vi "TIFFStream Write.vi"(7 "File data":T1, 8 "error in (no error)":errorcluster, 9 "Last image in file?":bool, 10 "Current and next IFD offset in":u32[](array[numeric]), 11 "Image data reference":refnum<data-value>) -> (0 "error out":errorcluster, 2 "Current and next IFD offset out":u32[](array[numeric]), 5 "File data out":T1)   [LabVIEW 2018]
uses:
  kernel32.dll
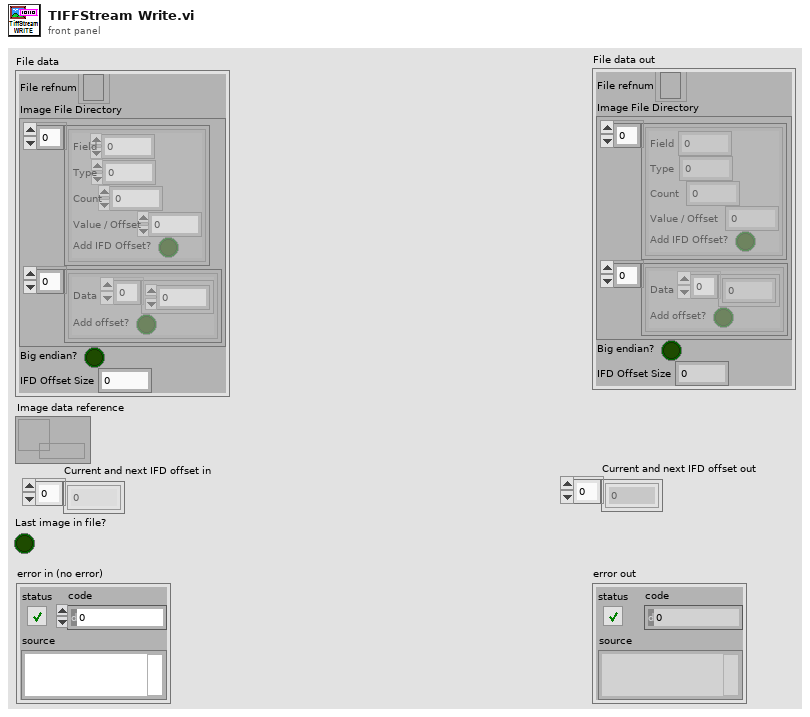
[diagram p1: front panel]
types:
  T1 = cluster{"File refnum":refnum<file>, "Image File Directory":cluster{cluster{"Field":u16, "Type":u16, "Count":u32, "Value / Offset":u32, "Add IFD Offset?":bool}[], cluster{"Data":u32[], "Add offset?":bool}[]}, "Big endian?":bool, "IFD Offset Size":u32}
  T2 = enum16{"big-endian, network order", "native, host order", "little-endian"}
  T3 = enum16{"open", "replace", "create", "open or create", "replace or create", "replace or create with confirmation"}
  T4 = cluster{cluster{"Field":u16, "Type":u16, "Count":u32, "Value / Offset":u32, "Add IFD Offset?":bool}[], cluster{"Data":u32[], "Add offset?":bool}[]}
  T5 = cluster{"Field":u16, "Type":u16, "Count":u32, "Value / Offset":u32, "Add IFD Offset?":bool}[]
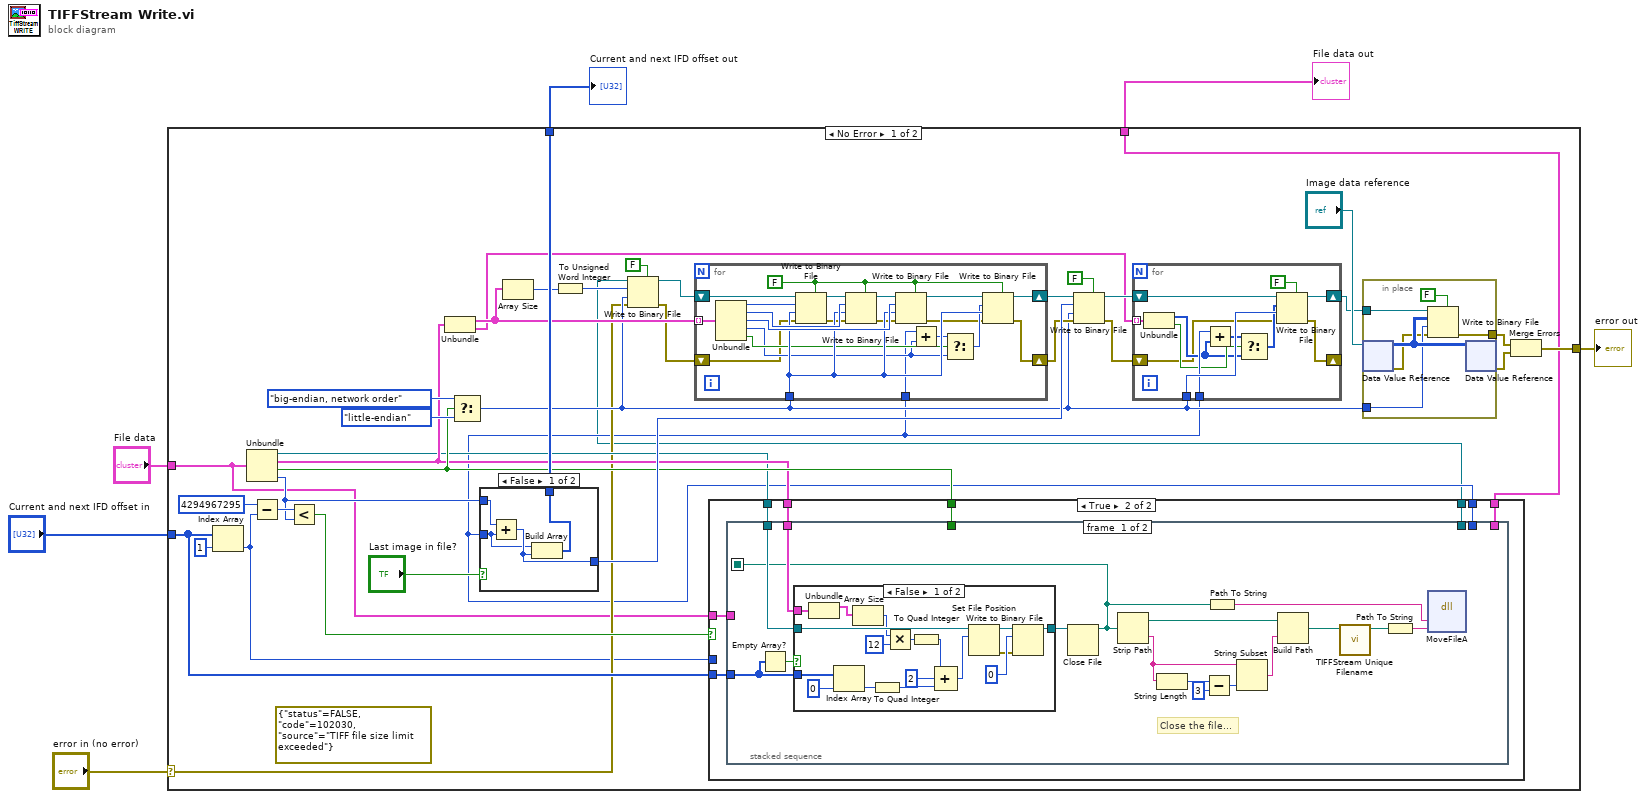
[diagram p0: block diagram]
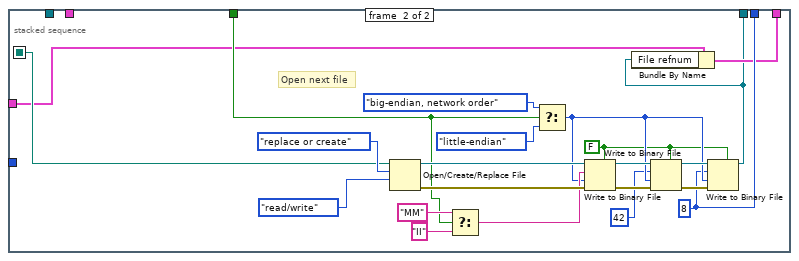
[diagram p4: hidden frame]
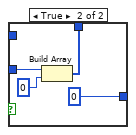
[diagram p5: hidden frame]
diagram:
  n1 = case shown="No Error" "error in (no error)" {
    selector: "error in (no error)" -> [w12 w160]
    tunnel: [w40 w160] -> w6
    tunnel: [w39 w161] -> w3
    tunnel: "Current and next IFD offset in" -> [w15 w161]
    tunnel: [w7 w159] -> w2
    tunnel: "File data" -> [w8 w159]
    frame No Error {
      (unwired) errorcluster {"status"=FALSE, "code"=102030, "source"="TIFF file size limit exceeded"} ("error IO")
      n2 = Index Array(array=w15, index=1) -> (element=w9:u32)
      n3 = Unbundle(w8) -> ("File refnum"=w16:refnum<file>, "Image File Directory"=w17:T4, "Big endian?"=w18:bool, "IFD Offset Size"=w36:u32)
      n4 = Subtract(x=u32 4294967295 ("IFD Offset"), y=w9) -> (x-y=w37:u32)
      n5 = Less?(x=w37, y=w36) -> (x < y?=w13:bool)
      n6 = Unbundle(w17) -> (w32:T5, w19:cluster{"Data":u32[], "Add offset?":bool}[])
      n7 = Select(t=T2."big-endian, network order" ("byte order (0:big-endian, network order)"), s=w18, f=T2."little-endian" ("byte order (0:big-endian, network order)")) -> (s? t:f=w22:T2)
      n8 = Array Size(array=w32) -> (size(s)=w31:i32)
      n9 = To Unsigned Word Integer(number=w31) -> (unsigned 16bit integer=w29:u16)
      n10 = case shown="True" w13 {
        tunnel: w18 -> [_ w55]
        tunnel: w17 -> [_ w54]
        tunnel: w16 -> [w47 w53]
        tunnel: w15 -> [_ w52]
        tunnel: [w46 w51] -> w11
        tunnel: [w47 w50] -> w10
        tunnel: w9 -> [w46 _]
        tunnel: w8 -> [w45 w49]
        tunnel: [w45 w48] -> w7
        frame False {
        }
        frame True {
          n11 = stacked-sequence {
            seq-local: [w58 _] -> [_ w94]
            tunnel: w55 -> [_ w95]
            tunnel: w54 -> [w71 _]
            tunnel: w53 -> [w70 _]
            tunnel: w52 -> [w59 _]
            tunnel: [_ w93] -> w51
            tunnel: [_ w90] -> w50
            tunnel: w49 -> [_ w92]
            tunnel: [_ w91] -> w48
            frame #0 {
              # "Close the file..."
              n12 = Empty Array?(array=w59) -> (empty?=w60:bool)
              n13 = case shown="False" w60 {
                tunnel: w70 -> [w88 w89]
                tunnel: w59 -> [w84 _]
                tunnel: w71 -> [w82 _]
                tunnel: [w72 w89] -> w61
                frame False {
                  n14 = Unbundle(w82) -> (w81:T5)  [unwired: 1 out]
                  n15 = Index Array(array=w84, index=0) -> (element=w86:u32)
                  n16 = Array Size(array=w81) -> (size(s)=w80:i32)
                  n17 = To Quad Integer(1:w86) -> (0:w85:i64)
                  n18 = Multiply(x=w80, y=12) -> (x*y=w77:i32)
                  n19 = To Quad Integer(1:w77) -> (0:w76:i64)
                  n20 = Compound Arithmetic op=ADD(w76, i64 2 ("x"), w85) -> (w83:i64)
                  n21 = Set File Position(offset (in bytes) (0)=w83, refnum=w88) -> (refnum out=w75:refnum<file>, error out=w73:errorcluster)  [unwired: 2 in]
                  n22 = Write to Binary File(file (use dialog)=w75, data=0, error in=w73) -> (refnum out=w72:refnum<file>)  [unwired: 3 in, 2 out]
                }
                frame True {
                }
              }
              n23 = Close File(refnum=w61) -> (path=w58:path)  [unwired: 1 in, 1 out]
              n24 = Strip Path(path=w58) -> (stripped path=w66:path, name=w65:string)
              n25 = String Length(string=w65) -> (length=w62:i32)
              n26 = Subtract(x=w62, y=3) -> (x-y=w64:i32)
              n27 = Path To String(path=w58) -> (string=w69:string)
              n28 = String Subset(string=w65, length (rest)=w64) -> (substring=w67:string)  [unwired: 1 in]
              n29 = Build Path(base path=w66, name or relative path=w67) -> (appended path=w57:path)
              n30 = call "TIFFStream Unique Filename.vi"("Path in"=w57) -> ("Unique path out"=w56:path)  [unwired: 10 in]
              n31 = Path To String(path=w56) -> (string=w68:string)
              n32 = dll-call lib="kernel32.dll" fn="MoveFileA"("arg1"=w69, "arg2"=w68) -> ()  [unwired: 6 in, 2 out]
            }
            frame #1 {
              w93 = u32 8
              w97 = FALSE ("prepend array or string size? (T)")
              # "Open next file"
              n33 = Open/Create/Replace File(file path (use dialog)=w94, operation (0:open)=T3."replace or create", access (0:read/write)=enum16{"read/write", "read-only", "write-only"}."read/write") -> (refnum out=w109:refnum<file>, error out=w106:errorcluster)  [unwired: 3 in, 1 out]
              n34 = Select(t="MM", s=w95, f="II") -> (s? t:f=w103:string)
              n35 = Select(t=T2."big-endian, network order" ("byte order (0:big-endian, network order)"), s=w95, f=T2."little-endian") -> (s? t:f=w98:T2)
              n36 = Write to Binary File(file (use dialog)=w109, data=w103, error in=w106, 5:w97, 9:w98) -> (refnum out=w100:refnum<file>, error out=w102:errorcluster)  [unwired: 1 in, 1 out]
              n37 = Write to Binary File(file (use dialog)=w100, data=u16 42, error in=w102, 5:w97, 9:w98) -> (refnum out=w99:refnum<file>, error out=w101:errorcluster)  [unwired: 1 in, 1 out]
              n38 = Write to Binary File(file (use dialog)=w99, data=w93, error in=w101, 5:w97, 9:w98) -> (refnum out=w90:refnum<file>)  [unwired: 1 in, 2 out]
              n39 = Bundle By Name(cluster=w92, "File refnum"=w90) -> (w91:T1)
            }
          }
        }
      }
      n40 = case shown="False" "Last image in file?" {
        tunnel: w11 -> [w145 w150]
        tunnel: [w146 u32 0] -> w34
        tunnel: w36 -> [w148 _]
        tunnel: [w147 w151] -> w39
        frame False {
          n41 = Add(x=w148, y=w145) -> (x+y=w146:u32)
          n42 = Build Array(w145, w146) -> (w147:u32[])
        }
        frame True {
          n43 = Build Array(w150, u32 0) -> (w151:u32[])
        }
      }
      n44 = Write to Binary File(file (use dialog)=w10, data=w29, error in=w12, 5:FALSE ("prepend array or string size? (T)"), 9:w22) -> (refnum out=w30:refnum<file>, error out=w28:errorcluster)  [unwired: 1 in, 1 out]
      n45 = for {
        tunnel: w32 -> [w144] mode=indexing
        tunnel: w22 -> [w135]
        tunnel: w11 -> [w130]
        shift-right: [w125] -> w25
        shift-left: w28 -> [w126]
        shift-right: [w124] -> w26
        shift-left: w30 -> [w138]
        w137 = FALSE ("prepend array or string size? (T)")
        n46 = Unbundle(w144) -> ("Field"=w143:u16, "Type"=w141:u16, "Count"=w139:u32, "Value / Offset"=w131:u32, "Add IFD Offset?"=w134:bool)
        n47 = Write to Binary File(file (use dialog)=w138, data=w143, error in=w126, 5:w137, 9:w135) -> (refnum out=w142:refnum<file>, error out=w129:errorcluster)  [unwired: 1 in, 1 out]
        n48 = Write to Binary File(file (use dialog)=w142, data=w141, error in=w129, 5:w137, 9:w135) -> (refnum out=w140:refnum<file>, error out=w128:errorcluster)  [unwired: 1 in, 1 out]
        n49 = Write to Binary File(file (use dialog)=w140, data=w139, error in=w128, 5:w137, 9:w135) -> (refnum out=w136:refnum<file>, error out=w127:errorcluster)  [unwired: 1 in, 1 out]
        n50 = Add(x=w130, y=w131) -> (x+y=w132:u32)
        n51 = Select(t=w132, s=w134, f=w131) -> (s? t:f=w133:u32)
        n52 = Write to Binary File(file (use dialog)=w136, data=w133, error in=w127, 5:w137, 9:w135) -> (refnum out=w124:refnum<file>, error out=w125:errorcluster)  [unwired: 1 in, 1 out]
      }
      n53 = Write to Binary File(file (use dialog)=w26, data=w34, error in=w25, 5:FALSE ("prepend array or string size? (T)"), 9:w22) -> (refnum out=w24:refnum<file>, error out=w23:errorcluster)  [unwired: 1 in, 1 out]
      n54 = for {
        tunnel: w19 -> [w123] mode=indexing
        tunnel: w22 -> [w121]
        tunnel: w11 -> [w118]
        shift-right: [w117] -> _
        shift-left: w23 -> [w114]
        shift-right: [w112] -> w21
        shift-left: w24 -> [w113]
        n55 = Unbundle(w123) -> ("Data"=w115:u32[], "Add offset?"=w116:bool)
        n56 = Add(x=w118, y=w115) -> (x+y=w119:u32[])
        n57 = Select(t=w119, s=w116, f=w115) -> (s? t:f=w120:u32[])
        n58 = Write to Binary File(file (use dialog)=w113, data=w120, error in=w114, 5:FALSE ("prepend array or string size? (T)"), 9:w121) -> (refnum out=w112:refnum<file>, error out=w117:errorcluster)  [unwired: 1 in, 1 out]
      }
      n59 = in-place {
        in-place-border: w21 -> [w154]
        in-place-border: w22 -> [w157]
        in-place-border: [w155] -> w42
        n60 = in-place-dvr #1("Image data reference") -> (w158:u16[][], w153:errorcluster)
        n61 = Write to Binary File(file (use dialog)=w154, data=w158, error in=w153, 5:FALSE ("prepend array or string size? (T)"), 9:w157) -> (error out=w155:errorcluster)  [unwired: 1 in, 2 out]
        n62 = in-place-dvr #1(w158) -> (w41:errorcluster)  [unwired: 1 out]
      }
      n63 = Merge Errors(w42, w41) -> (w40:errorcluster)
    }
    frame Error {
    }
  }
  "error out" <- w6
  "Current and next IFD offset out" <- w3
  "File data out" <- w2
